vi "4_3.vi"() -> ()   [LabVIEW 2022 SP3]
panel:
  out "Temperature History":cluster{dbl, "Temperature Value":dbl}(graph)
  in  "Stop Button":bool
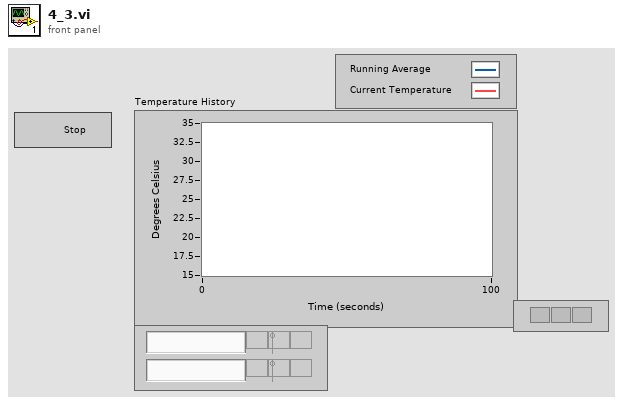
[diagram p1: front panel]
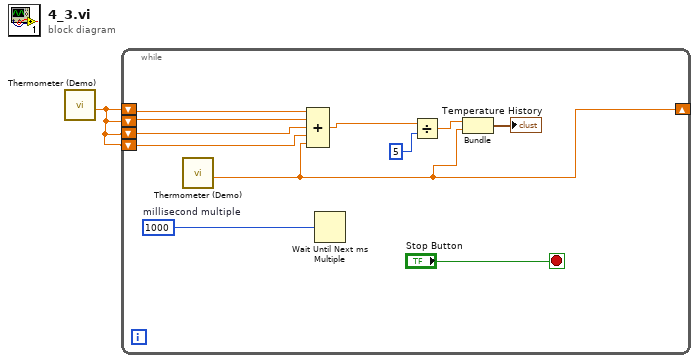
[diagram p0: block diagram]
diagram:
  n1 = call "Thermometer (Demo).vi"() -> ("Temperature Value"=w1:dbl)  [unwired: 11 in]
  n2 = while {
    shift-right: [w3] -> _
    shift-left: w1 -> [w10]
    shift-left: w1 -> [w9]
    shift-left: w1 -> [w8]
    shift-left: w1 -> [w7]
    stop <- "Stop Button" stop-if-true
    w12 = u32 1000  # millisecond multiple
    n3 = call "Thermometer (Demo).vi"() -> ("Temperature Value"=w3:dbl)  [unwired: 11 in]
    n4 = Compound Arithmetic op=ADD(w10, w9, w8, w7, w3) -> (w5:dbl)
    n5 = Wait Until Next ms Multiple(millisecond multiple=w12) -> ()  [unwired: 1 out]
    n6 = Divide(x=w5, y=5) -> (x/y=w4:dbl)
    n7 = Bundle(w4, "Temperature Value"=w3) -> (→"Temperature History":cluster{dbl, "Temperature Value":dbl})  [unwired: 1 in]
  }
